vi "ValueChange.vi"(0 "VI Reference In":refnum<vi>, 5 "Control Name":string, 7 "Value":variant, 11 "error in":errorcluster) -> (4 "VI Reference Out":refnum<vi>, 15 "error out":errorcluster)   [LabVIEW 2016]
doc: "This VI sets the value of top level controls in other VI"
uses:
  <vilib>/Utility/error.llb/Error Cluster From Error Code.vi
  <vilib>/ErrorRing/Error Ring.xnode
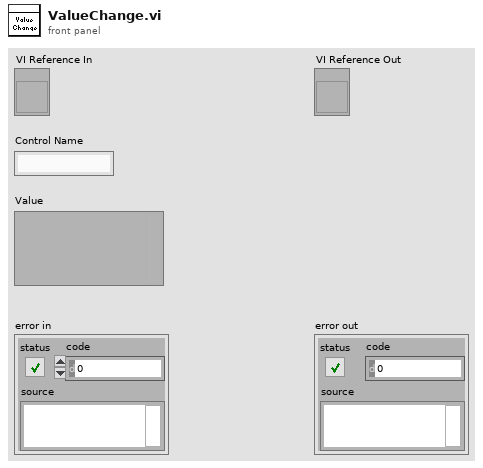
[diagram p1: front panel]
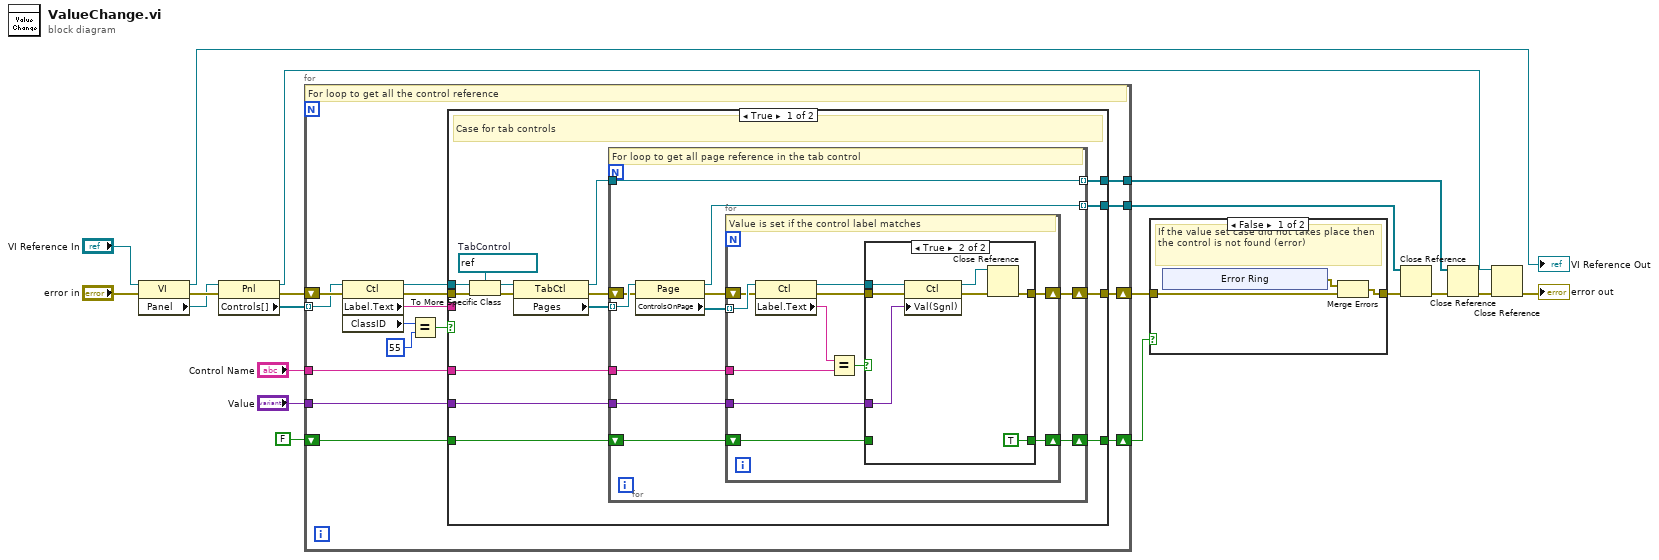
[diagram p0: block diagram]
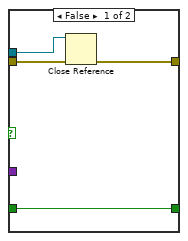
[diagram p3: hidden frame]
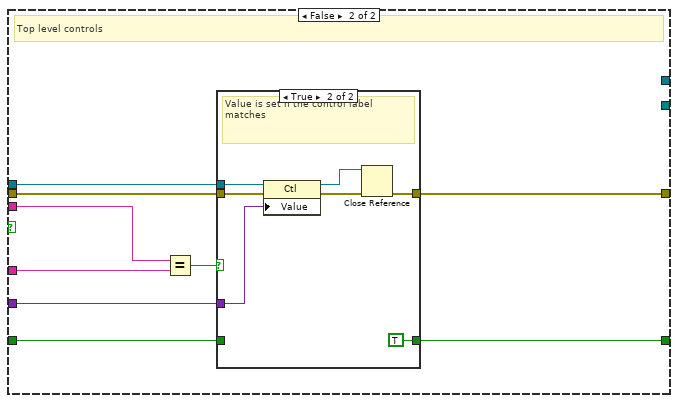
[diagram p4: hidden frame]
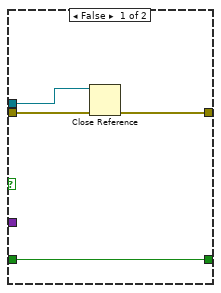
[diagram p5: hidden frame]
diagram:
  n1 = property class="VI"(reference="VI Reference In", error in="error in") -> (reference out=→"VI Reference Out":refnum<vi>, error out=w19:errorcluster, "Panel"=w15:refnum<vi>)
  n2 = property class="Pnl"(reference=w15, error in=w19) -> (reference out=w17:refnum<vi>, error out=w18:errorcluster, "Controls[]"=w14:refnum<vi>[])
  n3 = for {
    tunnel: w14 -> [w33] mode=indexing
    shift-right: [w31] -> w1
    shift-left: w18 -> [w34]
    tunnel: "Control Name" -> [w28]
    tunnel: "Value" -> [w27]
    tunnel: [w23] -> w8
    tunnel: [w22] -> w5
    shift-right: [w21] -> w3
    shift-left: FALSE -> [w20]
    # "For loop to get all the control reference"
    n4 = property class="Ctl"(reference=w33, error in=w34) -> (reference out=w30:refnum<vi>, error out=w32:errorcluster, "Label.Text"=w29:string, "ClassID"=w25:u32)
    n5 = Equal?(x=w25, y=u32 55) -> (x = y?=w26:bool)
    n6 = case shown="True" w26 {
      tunnel: w32 -> [w38 w91]
      tunnel: [w42 w90] -> w31
      tunnel: w30 -> [w44 w89]
      tunnel: w29 -> [_ w88]
      tunnel: w28 -> [w45 w87]
      tunnel: w27 -> [w46 w85]
      tunnel: [w41 _] -> w23
      tunnel: [w40 _] -> w22
      tunnel: [w36 w83] -> w21
      tunnel: w20 -> [w35 w84]
      frame True {
        w48 = refnum<vi> refnum  # TabControl
        # "Case for tab controls"
        n7 = To More Specific Class(target class=w48, reference=w44, error in=w38) -> (specific class reference=w49:refnum<vi>, error out=w37:errorcluster)
        n8 = property class="TabCtl"(reference=w49, error in=w37) -> (reference out=w39:refnum<vi>, error out=w43:errorcluster, "Pages"=w47:refnum<vi>[])
        n9 = for {
          tunnel: w47 -> [w59] mode=indexing
          tunnel: w46 -> [w58]
          tunnel: w45 -> [w57]
          shift-right: [w55] -> w42
          shift-left: w43 -> [w56]
          tunnel: [w53] -> w41 mode=indexing
          tunnel: [w52] -> w40 mode=indexing
          tunnel: w39 -> [w52]
          shift-right: [w51] -> w36
          shift-left: w35 -> [w50]
          # "For loop to get all page reference in the tab control"
          n10 = property class="Page"(reference=w59, error in=w56) -> (reference out=w53:refnum<vi>, error out=w54:errorcluster, "ControlsOnPage"=w60:refnum<vi>[])
          n11 = for {
            tunnel: w60 -> [w71] mode=indexing
            tunnel: w58 -> [w63]
            tunnel: w57 -> [w68]
            shift-right: [w65] -> w55
            shift-left: w54 -> [w64]
            shift-right: [w62] -> w51
            shift-left: w50 -> [w61]
            # "Value is set if the control label matches"
            n12 = property class="Ctl"(reference=w71, error in=w64) -> (reference out=w69:refnum<vi>, error out=w66:errorcluster, "Label.Text"=w67:string)
            n13 = Equal?(x=w67, y=w68) -> (x = y?=w70:bool)
            n14 = case shown="True" w70 {
              tunnel: w69 -> [w73 w82]
              tunnel: w66 -> [w75 w81]
              tunnel: [w74 w78] -> w65
              tunnel: w63 -> [_ w80]
              tunnel: [w72 TRUE] -> w62
              tunnel: w61 -> [w72 _]
              frame False {
                n15 = Close Reference(reference=w73, error in (no error)=w75) -> (error out=w74:errorcluster)
              }
              frame True {
                n16 = property class="Ctl"(reference=w82, error in=w81, "Val(Sgnl)"=w80) -> (reference out=w77:refnum<vi>, error out=w79:errorcluster)
                n17 = Close Reference(reference=w77, error in (no error)=w79) -> (error out=w78:errorcluster)
              }
            }
          }
        }
      }
      frame False {
        # "Top level controls"
        n18 = Equal?(x=w88, y=w87) -> (x = y?=w86:bool)
        n19 = case shown="True" w86 {
          tunnel: w91 -> [w95 w102]
          tunnel: [w94 w98] -> w90
          tunnel: w89 -> [w93 w101]
          tunnel: w85 -> [_ w100]
          tunnel: w84 -> [w92 _]
          tunnel: [w92 TRUE] -> w83
          frame False {
            n20 = Close Reference(reference=w93, error in (no error)=w95) -> (error out=w94:errorcluster)
          }
          frame True {
            # "Value is set if the control label matches"
            n21 = property class="Ctl"(reference=w101, error in=w102, "Value"=w100) -> (reference out=w97:refnum<vi>, error out=w99:errorcluster)
            n22 = Close Reference(reference=w97, error in (no error)=w99) -> (error out=w98:errorcluster)
          }
        }
      }
    }
  }
  n23 = case shown="False" w3 {
    tunnel: [w105 w111] -> w2
    tunnel: w1 -> [w104 w111]
    frame False {
      # "If the value set case did not takes place then the control is not found (error)"
      n24 = xnode "Error Ring"() -> ("error out"=w103:errorcluster)
      n25 = Merge Errors(w103, w104) -> (w105:errorcluster)
    }
    frame True {
      # "If the value set case takes place then the control is found (no error)"
    }
  }
  n26 = Close Reference(reference=w8, error in (no error)=w2) -> (error out=w7:errorcluster)
  n27 = Close Reference(reference=w5, error in (no error)=w7) -> (error out=w6:errorcluster)
  n28 = Close Reference(reference=w17, error in (no error)=w6) -> (error out=→"error out":errorcluster)
